vi "LED_Set.vi"(4 "RX":bool, 5 "RF":T1 items=["RF_0", "RF_1", "RF_2", "RF_3"], 6 "TX":bool, 7 "RFU":T2, 8 "Error_In":errorcluster, 10 "Auto_Sel_Rsrc?":bool=TRUE, 11 "VISA_Rsrc_In":refnum<visa-resource-name>) -> (0 "Error_Out":errorcluster, 3 "VISA_Rsrc_Out":refnum<visa-resource-name>)   [LabVIEW 2018]
uses:
  Types/RFU.ctl
  Types/RF.ctl
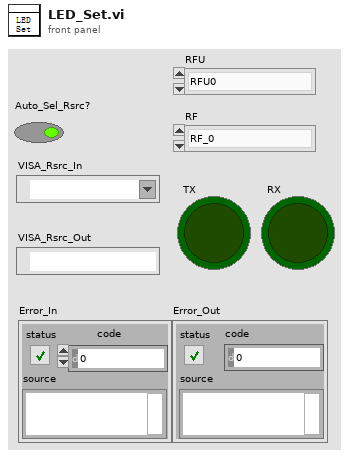
[diagram p1: front panel]
types:
  T1 = typedef "RF.ctl" = u16
  T2 = typedef "RFU.ctl" = enum8{"RFU0", "RFU1", "RFU2", "RFU3", "RFU4"}
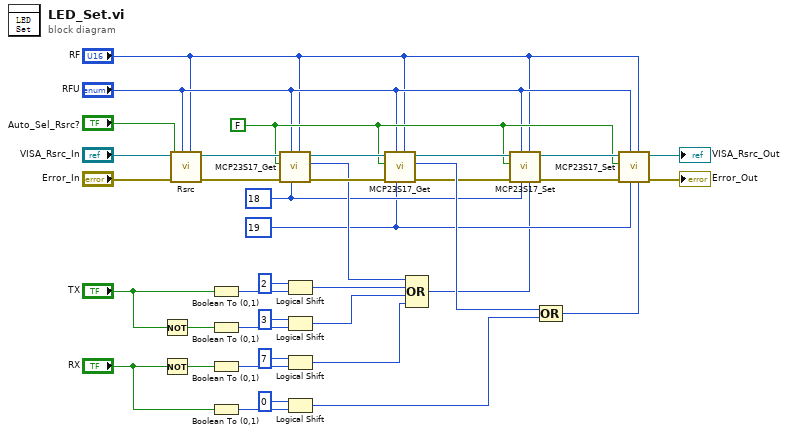
[diagram p0: block diagram]
diagram:
  w9 = FALSE ("Auto_Sel_Rsrc?")
  w5 = u32 19 ("Addr")
  w11 = u32 18 ("Addr")
  n1 = Not(x="TX") -> (.not. x?=w26:bool)
  n2 = Not(x="RX") -> (.not. x?=w21:bool)
  n3 = call "Rsrc.vi"("RF"="RF", "RFU"="RFU", "Error_In"="Error_In", "Auto_Sel_Rsrc?"="Auto_Sel_Rsrc?", "VISA_Rsrc_In"="VISA_Rsrc_In") -> ("Error_Out"=w35:errorcluster, "VISA_Rsrc_Out"=w36:refnum<visa-resource-name>)  [unwired: 5 in]
  n4 = Boolean To (0,1)(Boolean="TX") -> (0, 1=w29:i16)
  n5 = Boolean To (0,1)(Boolean=w26) -> (0, 1=w25:i16)
  n6 = Boolean To (0,1)(Boolean=w21) -> (0, 1=w23:i16)
  n7 = Boolean To (0,1)(Boolean="RX") -> (0, 1=w16:i16)
  n8 = call "MCP23S17_Get.vi"("RF"="RF", "Addr"=w11, "RFU"="RFU", "Error_In"=w35, "Auto_Sel_Rsrc?"=w9, "VISA_Rsrc_In"=w36) -> ("Error_Out"=w33:errorcluster, "Data"=w32:u32, "VISA_Rsrc_Out"=w34:refnum<visa-resource-name>)  [unwired: 3 in]
  n9 = Logical Shift(y=i16 2, x=w29) -> (x << y=w30:i16)
  n10 = Logical Shift(y=i16 3, x=w25) -> (x << y=w24:i16)
  n11 = Logical Shift(y=i16 7, x=w23) -> (x << y=w20:i16)
  n12 = Logical Shift(y=i16 0, x=w16) -> (x << y=w15:i16)
  n13 = call "MCP23S17_Get.vi"("RF"="RF", "Addr"=w5, "RFU"="RFU", "Error_In"=w33, "Auto_Sel_Rsrc?"=w9, "VISA_Rsrc_In"=w34) -> ("Error_Out"=w12:errorcluster, "Data"=w19:u32, "VISA_Rsrc_Out"=w14:refnum<visa-resource-name>)  [unwired: 3 in]
  n14 = Compound Arithmetic op=OR(w32, w30, w24, w20) -> (w2:u32)
  n15 = call "MCP23S17_Set.vi"("Data"=w2, "RF"="RF", "Addr"=w11, "RFU"="RFU", "Error_In"=w12, "Auto_Sel_Rsrc?"=w9, "VISA_Rsrc_In"=w14) -> ("Error_Out"=w8:errorcluster, "VISA_Rsrc_Out"=w10:refnum<visa-resource-name>)  [unwired: 3 in]
  n16 = Compound Arithmetic op=OR(w19, w15) -> (w1:u32)
  n17 = call "MCP23S17_Set.vi"("Data"=w1, "RF"="RF", "Addr"=w5, "RFU"="RFU", "Error_In"=w8, "Auto_Sel_Rsrc?"=w9, "VISA_Rsrc_In"=w10) -> ("Error_Out"=→"Error_Out":errorcluster, "VISA_Rsrc_Out"=→"VISA_Rsrc_Out":refnum<visa-resource-name>)  [unwired: 3 in]
